vi "Load Components.vi"(8 "error in (no error)":errorcluster, 10 "component names":string[](array[string]), 11 "Component Loader in":refnum<class "Component Loader.lvclass">) -> (0 "error out":errorcluster, 2 "Components":refnum<class "Component.lvclass">[](array[class]), 3 "Component Loader out":refnum<class "Component Loader.lvclass">)   [LabVIEW 2019, in "DSF Core.lvlib" / "Component Loader.lvclass"]
uses:
  Component Loader.lvclass
  Component/Component.lvclass
  Component/Component.lvclass/Component.ctl
  Component Loader.lvclass/Component Loader.ctl
  Find Packed Library.vi
  Load Classes.vi
  Find Packed Library Classes.vi
  Component Configuration/Find.vi
  Component User Interface/Find.vi
  Component/Default Buffer Converter/Create.vi
  Find Packed Libraries.vi
  Errors.vi
  Component Not Found.vi
  Load Class.vi
  <vilib>/Utility/error.llb/Clear Errors.vi
  New Component Loader Error.vi
  <vilib>/NI/Memory Manager/VIs/Write String to Source.vi
  Class Not Found.vi
  <vilib>/NI/Memory Manager/VIs/New Error Cluster.vi
  <vilib>/NI/Memory Manager/VIs/New Error Cluster (512B).vi
  Component Loader Error Info.vi
  <vilib>/NI/Memory Manager/VIs/Set Error Code.vi
  <vilib>/NI/Memory Manager/VIs/Set Error Status.vi
  <vilib>/NI/Memory Manager/VIs/Set Error Source.vi
  VIs/Constants/Constants.vi
  VIs/Constants/Engine Library Name.vi
  Base Error Offset.vi
  VIs/Constants/Base Error Code.vi
  Component/Default Buffer Converter/Default Buffer Converter Component.lvclass
  C:/Dev/GitHub/niveristand-data-sharing-framework-custom-device/Core/Classes/Component/Component.lvclass
  <vilib>/Utility/libraryn.llb/Recursive File List.vi
  <vilib>/Utility/LVLibp/Get Exported File List.vi
  <vilib>/Utility/libraryn.llb/Check if File or Folder Exists.vi
  <vilib>/Utility/LVClass/Get LV Class Default Value.vi
  Components/Buffer Converters/DSF Type Converter/Default Buffer Converter.lvclass
  Components/Buffer Converters/DSF Type Converter/User Interfaces/Default Buffer Converter User Interfaces.lvclass
  Components/Buffer Converters/DSF Type Converter/Configurations/Default Buffer Converter Configurations.lvclass
  Component User Interface/Component User Interfaces.lvclass
  Component Configuration/Component Configurations.lvclass
  DSF Core.lvlib
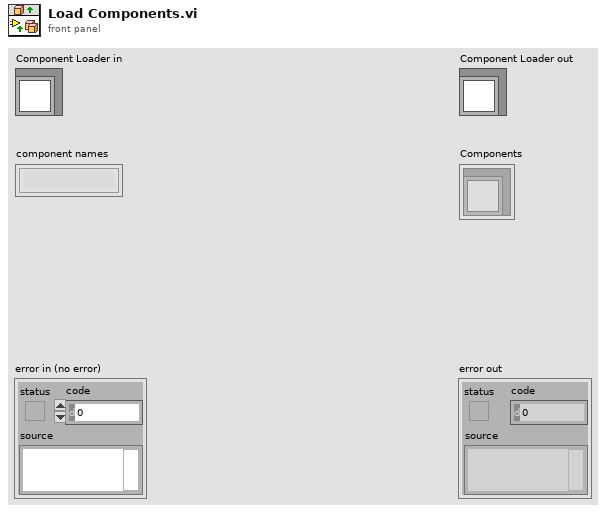
[diagram p1: front panel]
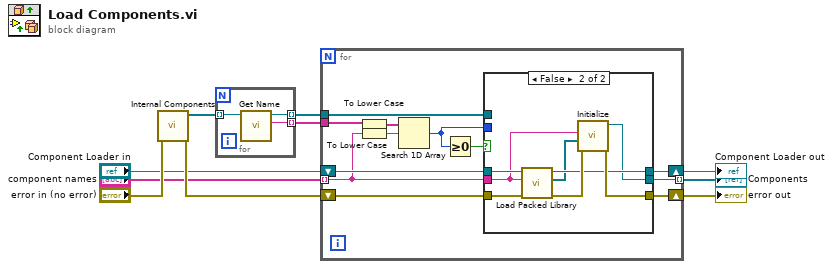
[diagram p0: block diagram]
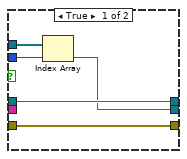
[diagram p2: hidden frame]
diagram:
  n1 = call "Internal Components.vi"("error in (no error)"="error in (no error)") -> ("error out"=w4:errorcluster, "Components"=w7:refnum<class "Component.lvclass">[])  [unwired: 9 in]
  n2 = for {
    tunnel: w7 -> [w13] mode=indexing
    tunnel: [w12] -> w1 mode=indexing
    tunnel: [w11] -> w6 mode=indexing
    n3 = call "Get Name.vi"("Component in"=w13) -> ("name"=w12:string, "Component out"=w11:refnum<class "Component.lvclass">)  [unwired: 9 in]
  }
  n4 = for {
    shift-right: [w22] -> w10
    shift-left: "Component Loader in" -> [w25]
    shift-right: [w23] -> w9
    shift-left: w4 -> [w24]
    tunnel: "component names" -> [w21] mode=indexing
    tunnel: w6 -> [w16]
    tunnel: [w17] -> w8 mode=indexing
    tunnel: w1 -> [w15]
    n5 = To Lower Case(string=w15) -> (all lower case string=w14:string[])
    n6 = To Lower Case(string=w21) -> (all lower case string=w18:string)
    n7 = Search 1D Array(1D array=w14, element=w18) -> (index of element=w19:i32)  [unwired: 1 in]
    n8 = Greater Or Equal To 0?(x=w19) -> (x >= 0?=w20:bool)
    n9 = case shown="False" w20 {
      tunnel: w25 -> [w30 w38]
      tunnel: w24 -> [w29 w37]
      tunnel: [w29 w35] -> w23
      tunnel: [w30 w34] -> w22
      tunnel: [w26 w33] -> w17
      tunnel: w21 -> [_ w31]
      tunnel: w16 -> [w28 _]
      tunnel: w19 -> [w27 _]
      frame True {
        n10 = Index Array(array=w28, index=w27) -> (element=w26:refnum<class "Component.lvclass">)
      }
      frame False {
        n11 = call "Load Packed Library.vi"("error in (no error)"=w37, "packed library name"=w31, "Component Loader in"=w38) -> ("error out"=w36:errorcluster, "objects"=w32:refnum<class>[], "Component Loader out"=w34:refnum<class "Component Loader.lvclass">)  [unwired: 6 in]
        n12 = call "Initialize.vi"("error in (no error)"=w36, "objects"=w32, "name"=w31) -> ("error out"=w35:errorcluster, "Component out"=w33:refnum<class "Component.lvclass">)  [unwired: 7 in]
      }
    }
  }
  "error out" <- w9
  "Component Loader out" <- w10
  "Components" <- w8
